vi "3D Ribbon Graph.vi"() -> ()   [LabVIEW 2020]
doc: "This VI shows how to use the 3D Ribbon Plot."
uses:
  <vilib>/Math Plots/3D Math Plots/3D Ribbon/3D Ribbon XCtrl/3D Ribbon.xctl
  <vilib>/Math Plots/3D Math Plots/3D Ribbon/3D Ribbon Datatype/Public/Plot Helper (Standard).vi
  <vilib>/Math Plots/3D Math Plots/3D Ribbon/3D Ribbon Datatype/3D Ribbon Datatype.lvclass
panel:
  out "3D Ribbon":refnum<class "3D Plot Datatype.lvclass">[](xcontrol)
  # "Overview: Demonstrates the Ribbon indicator from the Graph > 3D Graph palette.\nRequirements: LabVIEW Full Development System\nInstructions:\nRun the VI."
  # "Try the following operations on the graph:\n\n1. Click and drag the mouse within the graph to change the view direction.\n2. Press the Shift key and drag the mouse up to zoom in.\n3. Press the Shift key and drag the mouse down to zoom out.\n4. Right-click the graph and choose 3D Plot Properties to configure various properties related to the graph's appearance.\n5. Right-click the graph and select Export Image >Export to File."
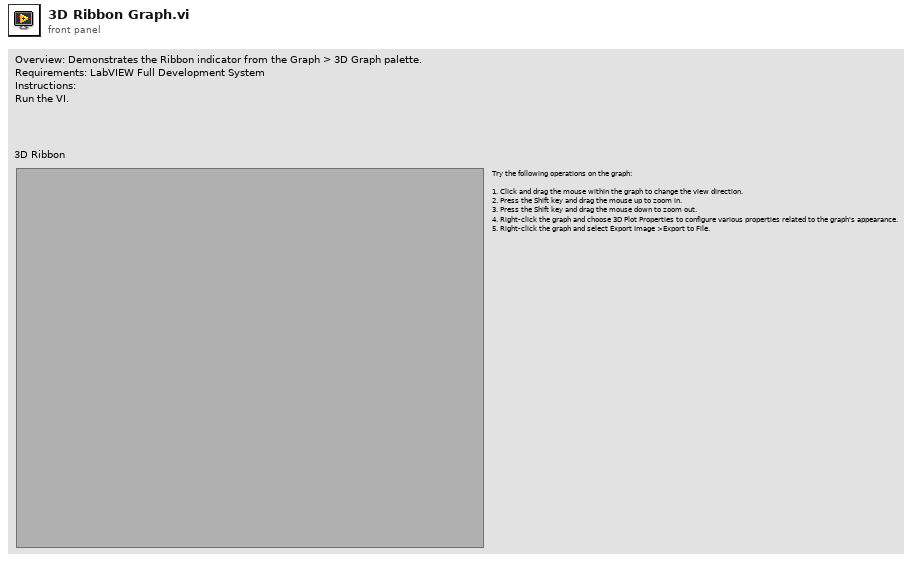
[diagram p1: front panel]
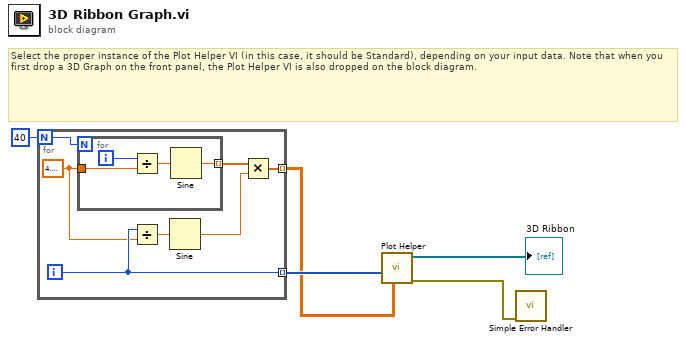
[diagram p0: block diagram]
diagram:
  # "Select the proper instance of the Plot Helper VI (in this case, it should be Standard), depending on your input data. Note that when you first drop a 3D Graph on the front panel, the Plot Helper VI is also dropped on the block diagram."
  n1 = for {
    N: 40 ("X input length") -> [w7]
    tunnel: [w9] -> w2 mode=indexing
    tunnel: [w8] -> w3 mode=indexing
    i -> [w8]
    w6 = sgl 4.2 ("y")
    n2 = for {
      N: w7 -> [_]
      tunnel: [w15] -> w11 mode=indexing
      tunnel: w6 -> [w13]
      i -> [w14]
      n3 = Divide(x=w14, y=w13) -> (x/y=w16:sgl)
      n4 = Sine(x=w16) -> (sin(x)=w15:sgl)
    }
    n5 = Divide(x=w8, y=w6) -> (x/y=w12:sgl)
    n6 = Sine(x=w12) -> (sin(x)=w10:sgl)
    n7 = Multiply(x=w11, y=w10) -> (x*y=w9:sgl[])
  }
  n8 = call-poly <vilib>:"Plot Helper.vi"("z matrix"=w2, "y vector"=w3) -> ("error out"=w1:errorcluster, "3D Plot lvclass Array out"=→"3D Ribbon":refnum<class "3D Plot Datatype.lvclass">[])  [unwired: 3 in, 5 out]
  n9 = call <vilib>:"Simple Error Handler.vi"("error in (no error)"=w1) -> ()  [unwired: 4 in, 5 out]
